vi "FP_Size Using Position and Bounds.vi"(6 "Border Spacing":i16, 8 "Error":errorcluster, 9 "Bounds":T3, 10 "Position":T2, 11 "VI":refnum<vi>) -> (0 "Error Out":errorcluster, 2 "Front Panel Box Out":T1, 3 "VI Out":refnum<vi>)   [LabVIEW 2025]
uses:
  <vilib>/Utility/miscctls.llb/LVBoundsTypeDef.ctl
  <vilib>/Utility/miscctls.llb/LVPositionTypeDef.ctl
  <vilib>/Utility/miscctls.llb/LVRectTypeDef.ctl
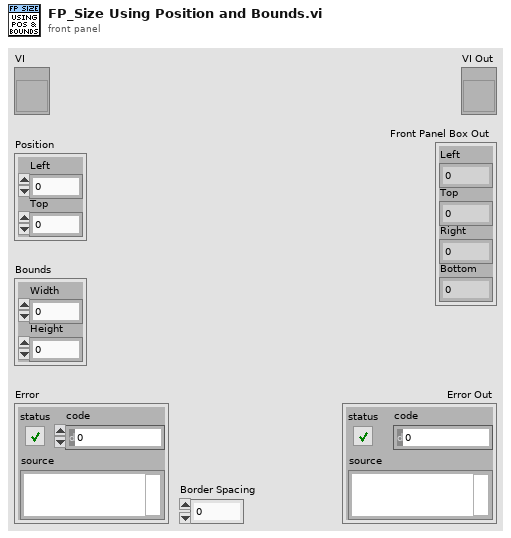
[diagram p1: front panel]
types:
  T1 = typedef "LVRectTypeDef.ctl" = cluster{"Left":i16, "Top":i16, "Right":i16, "Bottom":i16}
  T2 = typedef "LVPositionTypeDef.ctl" = cluster{"Left":i32, "Top":i32}
  T3 = typedef "LVBoundsTypeDef.ctl" = cluster{"Width":u32, "Height":u32}
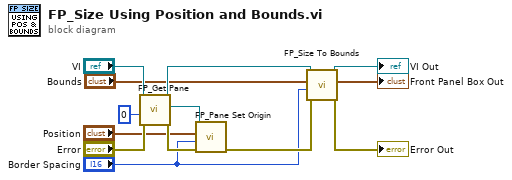
[diagram p0: block diagram]
diagram:
  n1 = call "FP_Get Pane.vi"("Error"="Error", "Pane Index"=0, "VI"="VI") -> ("Error Out"=w12:errorcluster, "Pane Refnum Out"=w13:refnum<vi>, "VI Out"=w9:refnum<vi>)  [unwired: 6 in]
  n2 = call "FP_Pane Set Origin.vi"("Error"=w12, "Border Spacing"="Border Spacing", "FP Position"="Position", "Pane"=w13) -> ("Error Out"=w6:errorcluster)  [unwired: 6 in, 1 out]
  n3 = call "FP_Size To Bounds.vi"("Error"=w6, "Border Spacing"="Border Spacing", "Bounds"="Bounds", "VI"=w9) -> ("Error Out"=→"Error Out":errorcluster, "Front Panel box"=→"Front Panel Box Out":T1, "VI Out"=→"VI Out":refnum<vi>)  [unwired: 5 in]
